vi "take from floor.vi"() -> ()   [LabVIEW 2018]
uses:
  vision/Vision info.vi
panel:
  in  "stop 2":bool
  in  "stop":bool
  out "Numeric":i32
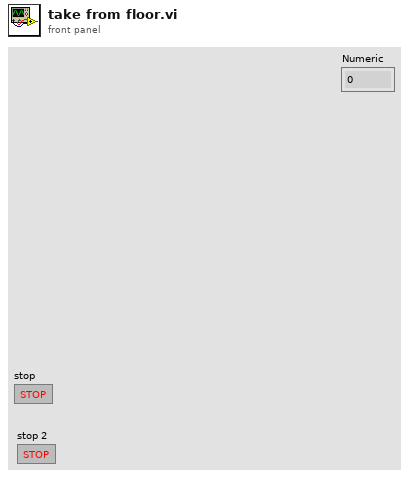
[diagram p1: front panel]
types:
  T1 = enum16{"shoulder", "elbow", "wrist", "base", "gripper"}
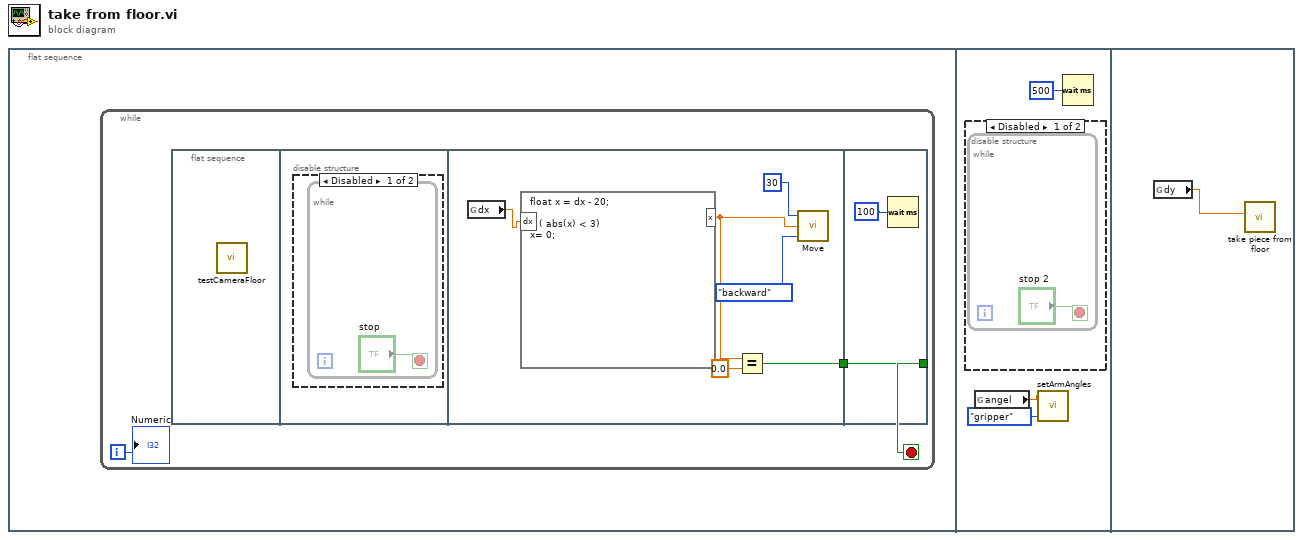
[diagram p0: block diagram]
diagram:
  n1 = flat-sequence {
    frame #0 {
      n2 = while {
        i -> [w2]
        stop <- w3 stop-if-true
        n3 = flat-sequence {
          tunnel: [w6] -> w1
          tunnel: [w12] -> w3
          tunnel: w1 -> [w12]
          frame #0 {
            n4 = call "testCameraFloor.vi"() -> ()  [unwired: 12 in]
          }
          frame #1 {
            n5 = disable-structure shown="Disabled" {
              frame Disabled {
                n6 = while {
                  stop <- "stop" stop-if-true
                }
              }
              frame Enabled {
              }
            }
          }
          frame #2 {
            n7 = global read "Vision info.vi" "dx"() -> (w5:dbl)
            n8 = formula code="float x = dx - 20;\n\nif ( abs(x) < 3)\nx= 0;"("dx"=w5) -> ("x"=w8:dbl)
            n9 = Equal?(x=w8, y=0.0) -> (x = y?=w6:bool)
            n10 = call "Move.vi"("Enum"=enum16{"forward", "backward", "left", "right"}."backward", "distance"=w8, "speed"=30) -> ()  [unwired: 1 in]
          }
          frame #3 {
            n11 = Wait (ms)(milliseconds to wait=u32 100) -> ()  [unwired: 1 out]
          }
        }
        "Numeric" <- w2
      }
    }
    frame #1 {
      n12 = disable-structure shown="Disabled" {
        frame Disabled {
          n13 = while {
            stop <- "stop 2" stop-if-true
          }
        }
        frame Enabled {
        }
      }
      n14 = global read "Vision info.vi" "angel"() -> (w14:dbl)
      n15 = call "setArmAngles.vi"("Enum"=T1."gripper", "angle"=w14) -> ()  [unwired: 2 in]
      n16 = Wait (ms)(milliseconds to wait=u32 500) -> ()  [unwired: 1 out]
    }
    frame #2 {
      n17 = global read "Vision info.vi" "dy"() -> (w17:dbl)
      n18 = call "take piece from floor.vi"("y"=w17) -> ()  [unwired: 11 in]
    }
  }
